vi "HookWindowProc.vi"(4 "error in (no error)":errorcluster, 6 "WindowProc\n(RESTORE)":T2, 7 "Window (\"\" - Parent)":string) -> (0 "error out":errorcluster, 2 "hWnd":T3, 3 "siwutil32":T1)   [LabVIEW 2011]
uses:
  siwutil32.ctl
  WinUSER/Windows/hWnd.ctl
  WINDOWPROCS.ctl
panel:
  in  "siwutil32":T1
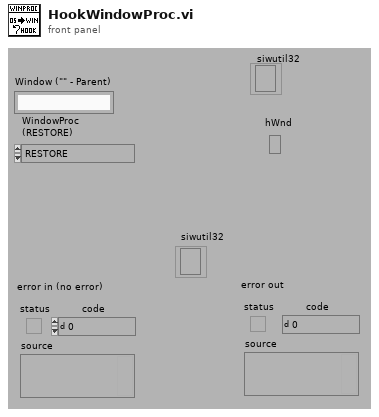
[diagram p1: front panel]
types:
  T1 = typedef "siwutil32.ctl" = refnum<k7>
  T2 = typedef "WINDOWPROCS.ctl" = enum16{"RESTORE"}
  T3 = typedef "hWnd.ctl" = refnum<k1>
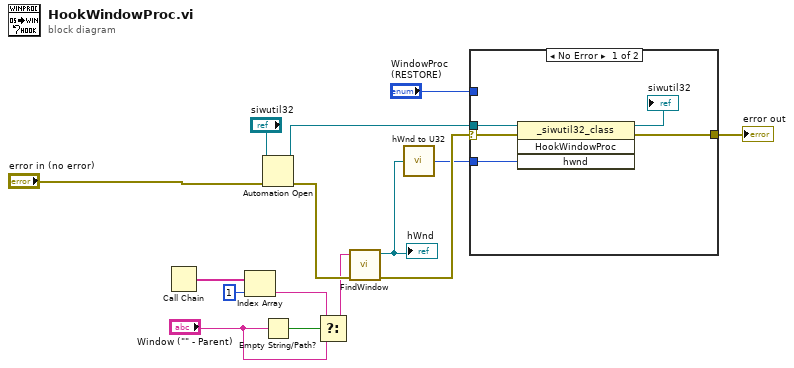
[diagram p0: block diagram]
diagram:
  n1 = Call Chain() -> (call chain=w12:string[])
  n2 = Index Array(array=w12, index=1) -> (element=w8:string)
  n3 = Automation Open(error in (no error)="error in (no error)", Automation Refnum="siwutil32") -> (Automation Refnum=w15:T1, error out=w13:errorcluster)  [unwired: 2 out]
  n4 = Empty String/Path?(string/path="Window (\"\" - Parent)") -> (empty?=w9:bool)
  n5 = Select(t=w8, s=w9, f="Window (\"\" - Parent)") -> (s? t:f=w6:string)
  n6 = call "FindWindow.vi"("error in (no error)"=w13, "window name (\"\")"=w6) -> ("error out"=w4:errorcluster, "hWnd"=w2:T3)  [unwired: 6 out]
  "hWnd" <- w2
  n7 = call "hWnd to U32.vi"("hWnd"=w2) -> ("hWnd"=w3:u32)  [unwired: 4 out]
  n8 = case shown="No Error" w4 {
    selector: w4 -> [w16 w21]
    tunnel: w15 -> [w20 _]
    tunnel: w3 -> [w19 _]
    tunnel: [w18 w21] -> w10
    tunnel: "WindowProc\n(RESTORE)" -> [_ _]
    frame No Error {
      n9 = invoke class="_siwutil32_class" method="HookWindowProc"(reference=w20, error in=w16, "hwnd"=w19) -> (reference out=→"siwutil32":T1, error out=w18:errorcluster)  [unwired: 1 in, 2 out]
    }
    frame Error {
    }
  }
  "error out" <- w10
